vi "huffman_decoder.vi"(8 "Python version":string, 9 "data_array_bit":i16[](array[numeric]), 10 "module path":path=path "D:/Thesis Pak Pri/huffman_decoder.vi", 11 "encode_array_bit":i32[](array[numeric])) -> (3 "return value":i32[](array[numeric]))   [LabVIEW 2018]
panel:
  out "error out":errorcluster
  in  "error in (no error)":errorcluster
  in  "function name":string="decode_huffman_image"
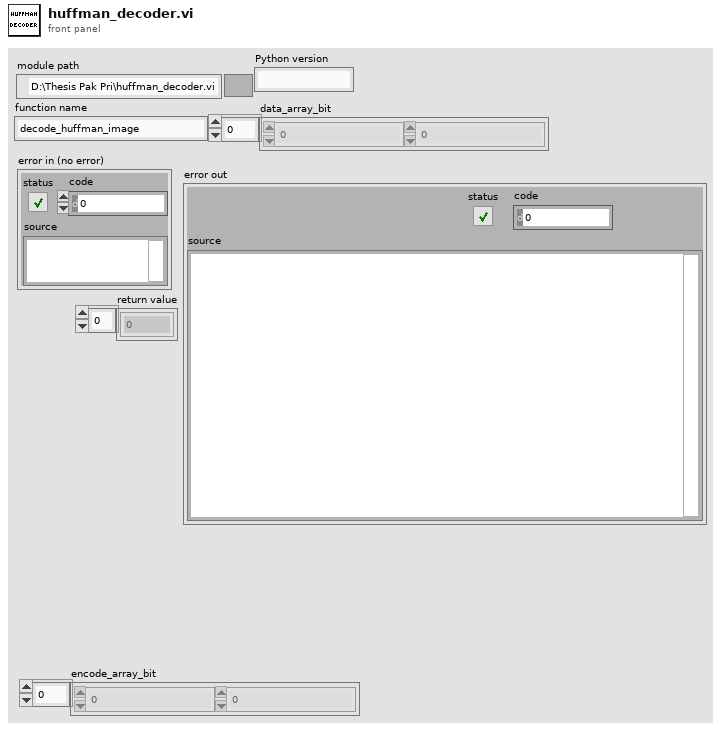
[diagram p1: front panel]
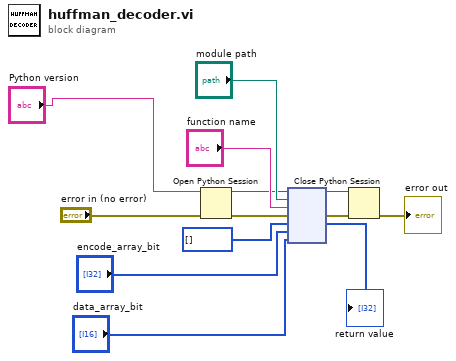
[diagram p0: block diagram]
diagram:
  n1 = Open Python Session(python version="Python version", 3:"error in (no error)") -> (session out=w11:refnum<k35>, error out=w10:errorcluster)  [unwired: 1 in]
  n2 = node(w11, "module path", "function name", w10, i32[] [], "encode_array_bit", "data_array_bit") -> (w9:refnum<k35>, w8:errorcluster, →"return value":i32[])  [unwired: 2 in, 2 out]
  n3 = Close Python Session(session in=w9, error in=w8) -> (11:→"error out":errorcluster)
